vi "Get Parameters from Hardware.vi"(8 "error in (no error)":errorcluster, 10 "Initial parameters":refnum<class "Mag Lab Parameters.lvclass">, 11 "Neocera in":refnum<class "Neocera.lvclass">) -> (0 "error out":errorcluster, 2 "Updated parameters":refnum<class "Mag Lab Parameters.lvclass">, 3 "Neocera out":refnum<class "Neocera.lvclass">)   [LabVIEW 2015, in "Neocera.lvclass"]
uses:
  Neocera.lvclass
  Mag Lab Properties/Mag Lab Parameters.lvclass
  NHMFL_Core/Libraries/Instruments/Temperature Controller/Controls/T controller parameters.ctl
  NHMFL_Core/Libraries/Instruments/Temperature Controller/Controls/Set Point Aproach.ctl
  Mag Lab Hardware.lvclass/Mag Lab Hardware.ctl
  Mag Lab Hardware.lvclass
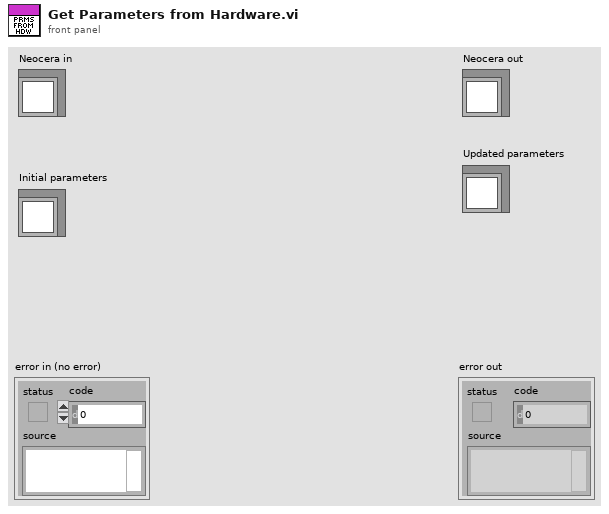
[diagram p1: front panel]
types:
  T1 = typedef "T controller parameters.ctl" = cluster{"Record heater":bool, "Record RAW":bool, "Set point":dbl, "Heater range":dbl, "Approach":T2, "Ramp rate, K/min":dbl, "Record Channels":string[], "Settling time ":dbl, "Settling range":dbl, "P":dbl, "I":dbl, "D":dbl, "Temperature Control":bool}
  T2 = typedef "Set Point Aproach.ctl" = enum16{"Instant", "Ramp"}
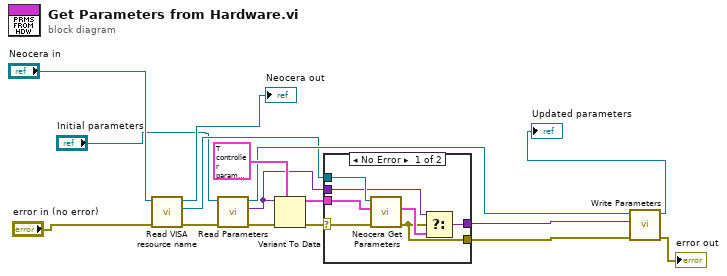
[diagram p0: block diagram]
diagram:
  n1 = call "Read VISA resource name.vi"("error in (no error)"="error in (no error)", "Mag Lab Hardware in"="Neocera in") -> ("error out"=w10:errorcluster, "VISA resource name"=w4:refnum<visa-resource-name>, "Mag Lab Hardware out"=→"Neocera out":refnum<class "Neocera.lvclass">)  [unwired: 7 in]
  n2 = call-dynamic "Read Parameters.vi"("error in (no error)"=w10, "Mag Lab Parameters in"="Initial parameters") -> ("error out"=w9:errorcluster, "Parameters"=w12:variant, "Mag Lab Parameters out"=w11:refnum<class "Mag Lab Parameters.lvclass">)  [unwired: 7 in]
  n3 = Variant To Data(error in=w9, type=T1 {"Record heater"=FALSE, "Record RAW"=FALSE, "Set point"=0.0, "Heater range"=0.0, "Approach"=enum."Instant", "Ramp rate, K/min"=0.0, "Record Channels"=[], "Settling time "=60.0, "Settling range"=0.1, "P"=0.0, "I"=0.0, "D"=0.0, "Temperature Control"=FALSE} ("Data"), Variant=w12) -> (data=w13:T1, error out=w14:errorcluster)
  n4 = case shown="No Error" w14 {
    selector: w14 -> [w22 _]
    tunnel: w13 -> [w23 _]
    tunnel: [w18 w24] -> w16
    tunnel: w12 -> [w20 w24]
    tunnel: w4 -> [w21 _]
    tunnel: [w17 _] -> w8
    frame No Error {
      n5 = call "Neocera Get Parameters.vi"("error in (no error)"=w22, "Control Panel Data"=w23, "VISA resource name"=w21) -> ("error out"=w17:errorcluster, "Control Panel Data Out"=w19:T1)  [unwired: 6 in, 1 out]
      n6 = Select(t=w20, s=w17, f=w19) -> (s? t:f=w18:variant)
    }
    frame Error {
    }
  }
  n7 = call-dynamic "Write Parameters.vi"("error in (no error)"=w8, "Parameters"=w16, "Mag Lab Parameters in"=w11) -> ("error out"=→"error out":errorcluster, "Mag Lab Parameters out"=→"Updated parameters":refnum<class "Mag Lab Parameters.lvclass">)  [unwired: 7 in]
